vi "Event Handler.vi"(8 "error in (no error)":errorcluster, 10 "Stop Event Handler":refnum<user-event>, 11 "TreeDirectory in":refnum<class "TreeDirectoryExt.lvclass">) -> (0 "error out":errorcluster)   [LabVIEW 2025, in "TreeDirectoryExt.lvclass"]
doc: "The <b>Event Handler VI</b> is a dynamic dispatch VI that should be overwritten if events are needed to create the enhanced QControl. \n\nBy inheriting from the main Control.lvclass the overwritten <b>Event Handler VI</b> will be launched asynchronously in the initialization of the QControl.\n<b> </b> <b> </b>\n©2016 Q Software Innovations, LLC (QSI)\nwritten by Quentin Alldredge\nproduced in LabVIEW 2015\n\nsupport@qsoftwareinnovations.com\nwww.qsoftwareinnovations.com\n\nAll rights reserved.\n\nRedistribution and use in source and binary forms, with or without modification, are permitted provided that the following conditions are met:\n\n * Redistributions of source code must retain the above copyright notice, this list of conditions and the following disclaimer.\n * Redistributions in binary form must reproduce the above copyright notice, this list of conditions and the following disclaimer in the documentation and/or other materials provided with the distribution.\n * Neither the name of Q Software Innovations, LLC. nor the names of its contributors may be used to endorse or promote products derived from this software without specific prior written permission.\n\nTHIS SOFTWARE IS PROVIDED BY THE COPYRIGHT HOLDERS AND CONTRIBUTORS \"AS IS\" AND ANY EXPRESS OR IMPLIED WARRANTIES, INCLUDING, BUT NOT LIMITED TO, THE IMPLIED WARRANTIES OF MERCHANTABILITY AND FITNESS FOR A PARTICULAR PURPOSE ARE DISCLAIMED. IN NO EVENT SHALL THE COPYRIGHT OWNER OR CONTRIBUTORS BE LIABLE FOR ANY DIRECT, INDIRECT, INCIDENTAL, SPECIAL, EXEMPLARY, OR CONSEQUENTIAL DAMAGES (INCLUDING, BUT NOT LIMITED TO, PROCUREMENT OF SUBSTITUTE GOODS OR SERVICES; LOSS OF USE, DATA, OR PROFITS; OR BUSINESS INTERRUPTION) HOWEVER CAUSED AND ON ANY THEORY OF LIABILITY, WHETHER IN CONTRACT, STRICT LIABILITY, OR TORT (INCLUDING NEGLIGENCE OR OTHERWISE) ARISING IN ANY WAY OUT OF THE USE OF THIS SOFTWARE, EVEN IF ADVISED OF THE POSSIBILITY OF SUCH DAMAGE."
uses:
  TreeDirectoryExt.lvclass
  TreeDirectoryExt.lvclass/TreeDirectoryExt.ctl
  <vilib>/QSI/QControls/QControl Classes/TreeControl/TreeControl.lvclass
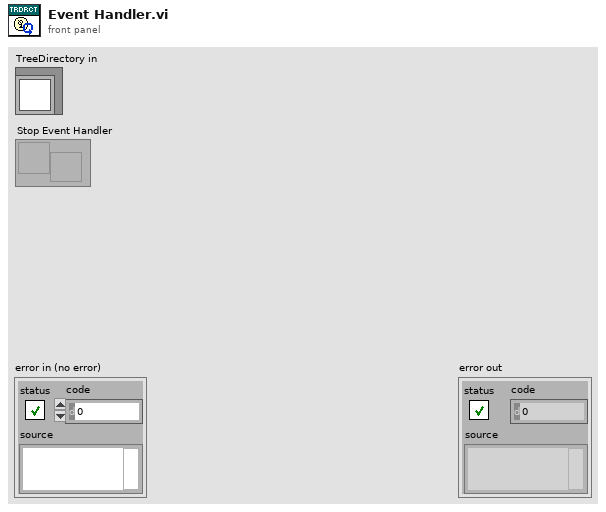
[diagram p1: front panel]
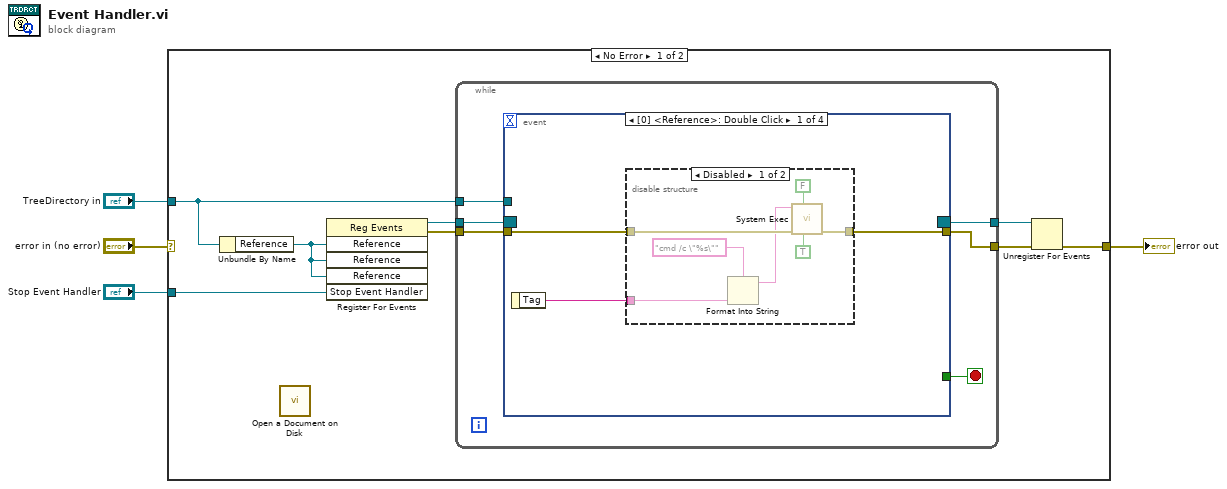
[diagram p0: block diagram]
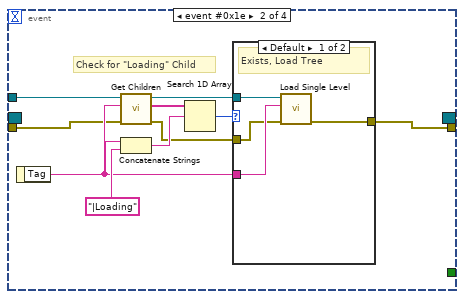
[diagram p3: hidden frame]
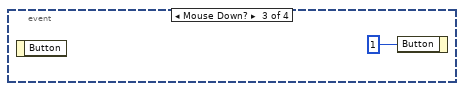
[diagram p5: hidden frame]
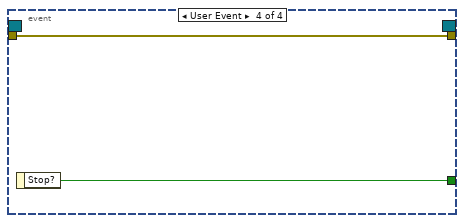
[diagram p6: hidden frame]
diagram:
  n1 = case shown="No Error" "error in (no error)" {
    selector: "error in (no error)" -> [_ w48]
    tunnel: [w9 w48] -> w3
    tunnel: "TreeDirectory in" -> [w7 _]
    tunnel: "Stop Event Handler" -> [w6 _]
    frame No Error {
      n2 = Unbundle By Name(w7) -> ("Reference"=w5:refnum<vi>)
      n3 = call <vilib>:"Open a Document on Disk.vi"() -> ()  [unwired: 7 in, 1 out]
      n4 = register-events(w5, w5, w5, w6) -> (reference out=w12:refnum<event-registration>, error out=w11:errorcluster)  [unwired: 2 in]
      n5 = while {
        tunnel: w12 -> [w18]
        tunnel: w11 -> [w16]
        tunnel: [w15] -> w10
        tunnel: [w13] -> w8
        tunnel: w7 -> [w17]
        stop <- w14 stop-if-true
        n6 = event shown="[0] <Reference>: Double Click" {
          selector: w18 -> [_ _ _ _]
          dyn-events: [_ _ _ _] -> w13
          timeout: _ -> [_ _ _ _]
          tunnel: w17 -> [_ w39 _ _]
          tunnel: w16 -> [w21 w32 _ w47]
          tunnel: [w20 w30 _ w47] -> w15
          tunnel: [_ _ _ w46] -> w14
          event Double Click {
            n7 = event-data() -> ("Tag"=w19:string)  [unwired: 1 in]
            n8 = disable-structure shown="Disabled" {
              disable-tunnel: w21 -> [w28 w29]
              disable-tunnel: [w27 w29] -> w20
              disable-tunnel: w19 -> [w26 _]
              frame Disabled {
                n9 = Format Into String(format string="cmd /c \"%s\"", w26) -> (resulting string=w24:string)  [unwired: 2 in, 1 out]
                n10 = call <vilib>:"System Exec.vi"("run minimized? (F)"=TRUE, "wait until completion? (T)"=FALSE, "error in (no error)"=w28, "command line"=w24) -> ("error out"=w27:errorcluster)  [unwired: 4 in, 3 out]
              }
              frame Enabled {
              }
            }
          }
          event event #0x1e {
            # "Check for \"Loading\" Child"
            n11 = event-data() -> ("Tag"=w33:string)  [unwired: 1 in]
            n12 = call <vilib>:"Get Children.vi"("error in (no error)"=w32, "Tag"=w33, "Tree in"=w39) -> ("error out"=w31:errorcluster, "ChildrenTags[]"=w37:string[], "Tree out"=w34:refnum<class "TreeDirectoryExt.lvclass">)  [unwired: 6 in]
            n13 = Concatenate Strings(w33, "|Loading" ("string")) -> (w36:string)
            n14 = Search 1D Array(1D array=w37, element=w36) -> (index of element=w35:i32)  [unwired: 1 in]
            n15 = case shown="Default" w35 {
              tunnel: w34 -> [w43 _]
              tunnel: w33 -> [w42 _]
              tunnel: w31 -> [w41 w44]
              tunnel: [w40 w44] -> w30
              frame Default {
                # "Exists, Load Tree"
                n16 = call "Load Single Level.vi"("error in (no error)"=w41, "Tag"=w42, "TreeDirectory in"=w43) -> ("error out"=w40:errorcluster)  [unwired: 7 in, 1 out]
              }
              frame -1 {
                # "DNE, Do Nothing"
              }
            }
          }
          event Mouse Down? {
            n17 = event-data() -> ()  [unwired: 1 in, 1 out]
            n18 = event-data("Button"=u16 1) -> ()  [unwired: 1 in, 1 out]
          }
          event User Event {
            n19 = event-data() -> ("Stop?"=w46:bool)  [unwired: 1 in]
          }
        }
      }
      n20 = Unregister For Events(event registration refnum=w8, error in=w10) -> (error out=w9:errorcluster)
    }
    frame Error {
    }
  }
  "error out" <- w3
